vi "Validate.vi"(8 "error in (no error)":errorcluster, 11 "Build in":refnum<class "AB_WebService.lvclass">) -> (0 "error out":errorcluster, 3 "Build out":refnum<class "AB_WebService.lvclass">)   [LabVIEW 2020, in "AB_WebService.lvclass"]
uses:
  <vilib>/AppBuilder/AB_Classes/WebService/AB_WebService.lvclass
  <vilib>/AppBuilder/AB_Source_Inclusion.ctl
  <resource>/Framework/Providers/Common/provcom_StringGlobals.vi
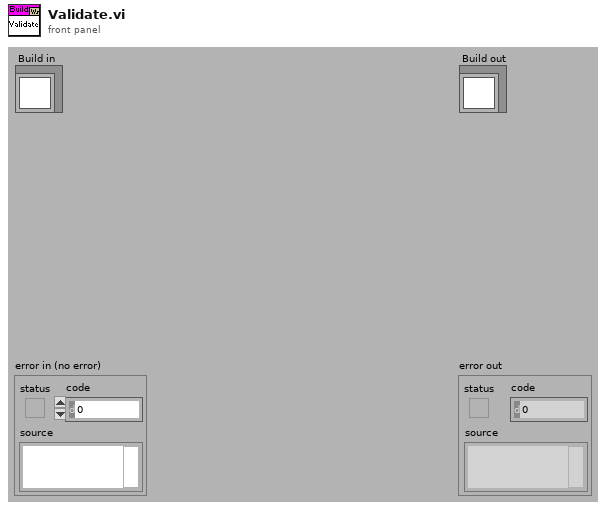
[diagram p1: front panel]
types:
  T1 = typedef "AB_Source_Inclusion.ctl" = enum16{"IncludeIfReferenced", "Include", "Exclude", "TopLevel"}
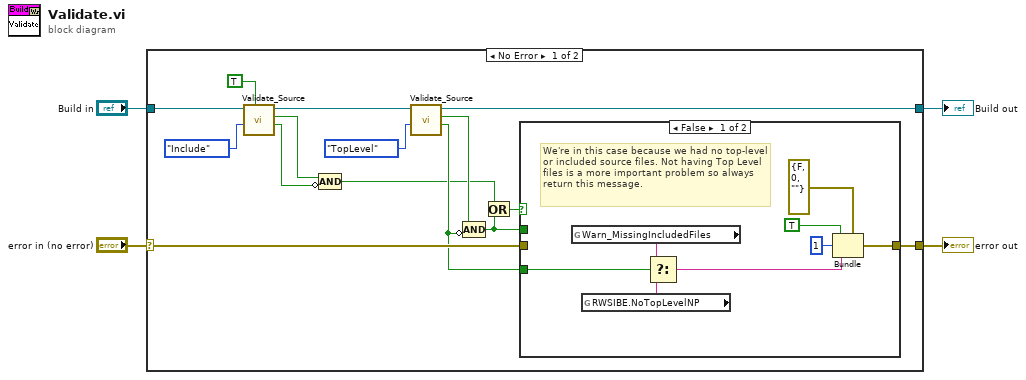
[diagram p0: block diagram]
diagram:
  n1 = case shown="No Error" "error in (no error)" {
    selector: "error in (no error)" -> [w17 w30]
    tunnel: [w16 w30] -> w1
    tunnel: [w19 w29] -> w3
    tunnel: "Build in" -> [w14 w29]
    frame No Error {
      n2 = call-dynamic "Validate_Source.vi"("check non-TopLevel"=TRUE, "sourceInclusion"=AB_Source_Inclusion."Include", "AB_Build in"=w14) -> ("missingFiles"=w5:bool, "includedFiles"=w9:bool, "AB_Build out"=w13:refnum<class "AB_WebService.lvclass">)  [unwired: 4 in, 2 out]
      n3 = Compound Arithmetic op=AND(w9, invert w5) -> (w6:bool)
      n4 = call-dynamic "Validate_Source.vi"("sourceInclusion"=AB_Source_Inclusion."TopLevel", "AB_Build in"=w13) -> ("missingFiles"=w15:bool, "includedFiles"=w10:bool, "AB_Build out"=w19:refnum<class "AB_WebService.lvclass">)  [unwired: 5 in, 2 out]
      n5 = Compound Arithmetic op=AND(w10, invert w15) -> (w7:bool)
      n6 = Or(x=w6, y=w7) -> (x .or. y?=w8:bool)
      n7 = case shown="False" w8 {
        tunnel: [w24 w28] -> w16
        tunnel: w17 -> [_ w28]
        tunnel: w15 -> [w23 _]
        tunnel: w7 -> [_ _]
        frame False {
          # "We're in this case because we had no top-level or included source files. Not having Top Level files is a more important problem so always return this message."
          n8 = global read "provcom_StringGlobals.vi" "Warn_MissingIncludedFiles"() -> (w21:string)
          n9 = global read "provcom_StringGlobals.vi" "RWSIBE.NoTopLevelNP"() -> (w20:string)
          n10 = Select(t=w21, s=w23, f=w20) -> (s? t:f=w22:string)
          n11 = Bundle(cluster=errorcluster {"status"=FALSE, "code"=0, "source"=""} ("error IO"), "status"=TRUE, "code"=1, "source"=w22) -> (w24:errorcluster)
        }
        frame True {
          # "As long as some files are included in the build, this check passes. Not having Top level VIs is ok since it's possible to have a web service that only contains static documents."
        }
      }
    }
    frame Error {
    }
  }
  "error out" <- w1
  "Build out" <- w3
